vi "719 Get Devices Info From DB.vi"(8 "error in (no error)":errorcluster caption="错误输入（无错误）") -> (0 "error out":errorcluster caption="错误输出", 1 "Type":string[](array[string]), 2 "IP Address":string[](array[string]), 3 "Device Name":string[](array[string]))   [LabVIEW 2018]
uses:
  <vilib>/drjdpowell/SQLite Library/SQL Connection/Connection.lvclass
  <vilib>/drjdpowell/SQLite Library/SQL Connection/Open (path).vi
  <vilib>/drjdpowell/SQLite Library/SQL Connection/Open (string).vi
  <vilib>/AdvancedString/Path To Command Line String.vi
  <vilib>/drjdpowell/SQLite Library/SQL Connection/Execute SQL.vi
  <vilib>/drjdpowell/SQLite Library/SQLite.lvlib
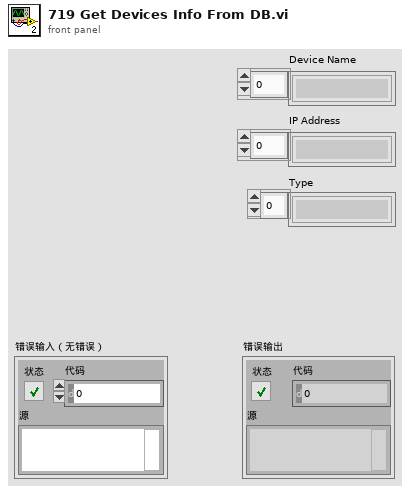
[diagram p1: front panel]
types:
  T1 = enum16{"New or existing", "Existing", "Read only"}
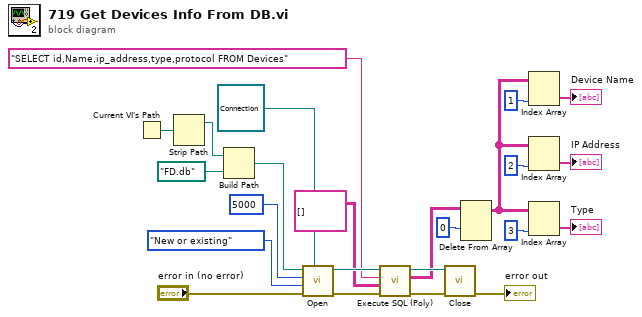
[diagram p0: block diagram]
diagram:
  n1 = Current VI's Path() -> (path=w21:path)
  n2 = Strip Path(path=w21) -> (stripped path=w20:path)  [unwired: 1 out]
  n3 = Build Path(base path=w20, name or relative path=path "FD.db" ("template (empty)")) -> (appended path=w19:path)
  n4 = call-poly <vilib>:"Open.vi"("SQLite Connection type"=refnum<class "Connection.lvclass"> refnum, "error in (no error)"="error in (no error)", "File Option"=T1."New or existing", "busy timeout (ms)"=5000, "db file"=w19) -> ("error out"=w14:errorcluster, "SQLite Connection"=w17:refnum<class "Connection.lvclass">)  [unwired: 5 in]
  n5 = call-poly <vilib>:"Execute SQL (Poly).vi"("error in (no error)"=w14, "Default Result"=string[][] [], "SQL"="SELECT id,Name,ip_address,type,protocol FROM Devices", "SQLite Connection in"=w17) -> ("error out"=w15:errorcluster, "Result Set"=w6:string[][], "SQLite Connection"=w16:refnum<class "Connection.lvclass">)  [unwired: 4 in, 1 out]
  n6 = call-dynamic "Close.vi"("error in (no error)"=w15, "SQLite Connection in"=w16) -> ("error out"=→"error out":errorcluster)  [unwired: 9 in]
  n7 = Delete From Array(array=w6, index (row)=0 ("索引")) -> (array with subset deleted=w4:string[][])  [unwired: 2 in, 1 out]
  n8 = Index Array(array=w4, index (col)=1 ("禁用的索引 (列)")) -> (element=→"Device Name":string[])  [unwired: 1 in]
  n9 = Index Array(array=w4, index (col)=2 ("禁用的索引 (列)")) -> (element=→"IP Address":string[])  [unwired: 1 in]
  n10 = Index Array(array=w4, index (col)=3 ("禁用的索引 (列)")) -> (element=→"Type":string[])  [unwired: 1 in]
